vi "Test Case, Charging State Color.vi"() -> ()   [LabVIEW 2010]
panel:
  in  "ChargingState 7":string="zzzz"
  in  "ChargingState 6":string="CHARGE_ERROR-5"
  in  "ChargingState 5":string="CHARGE_COMPLETE-4"
  in  "ChargingState 4":string="CHARGE_CC_SLOW-3"
  in  "ChargingState 3":string="CHARGE_CC_FAST-2"
  in  "ChargingState 2":string="CHARGE_PRE_CONDITION-1"
  in  "ChargingState":string="CHARGE_OFF-0"
  in  "error in":errorcluster
  out "error out":errorcluster
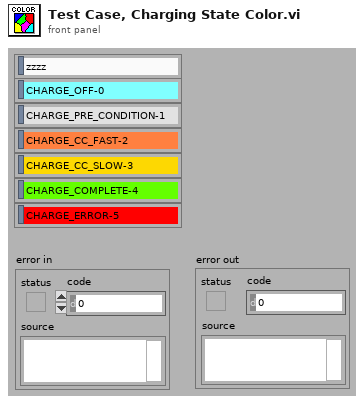
[diagram p1: front panel]
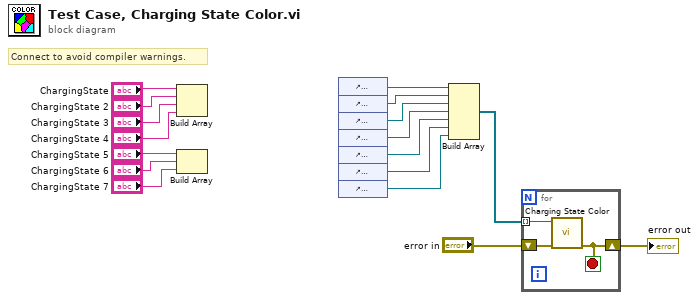
[diagram p0: block diagram]
diagram:
  # "Connect to avoid compiler warnings."
  n1 = Build Array("ChargingState", "ChargingState 2", "ChargingState 3", "ChargingState 4") -> ()  [unwired: 1 out]
  n2 = Build Array("ChargingState 5", "ChargingState 6", "ChargingState 7") -> ()  [unwired: 1 out]
  n3 = control-ref of="ChargingState"() -> (w17:refnum<vi>)
  n4 = control-ref of="ChargingState 2"() -> (w16:refnum<vi>)
  n5 = control-ref of="ChargingState 3"() -> (w15:refnum<vi>)
  n6 = control-ref of="ChargingState 4"() -> (w14:refnum<vi>)
  n7 = control-ref of="ChargingState 5"() -> (w13:refnum<vi>)
  n8 = control-ref of="ChargingState 6"() -> (w12:refnum<vi>)
  n9 = control-ref of="ChargingState 7"() -> (w11:refnum<vi>)
  n10 = Build Array(w17, w16, w15, w14, w13, w12, w11) -> (w10:refnum<vi>[])
  n11 = for {
    tunnel: w10 -> [w20] mode=indexing
    shift-right: [w19] -> w9
    shift-left: "error in" -> [w18]
    stop <- w19 stop-if-true
    n12 = call "Charging State Color.vi"("error in"=w18, "Str Refnum"=w20) -> ("error out"=w19:errorcluster)  [unwired: 5 in]
  }
  "error out" <- w9
